vi "Auton Go Backwards.vi"(7 "output range":cluster{"output high":dbl, "output low":dbl}, 9 "Goal":dbl, 10 "PID setpoint":dbl, 11 "Average gains":T1) -> (2 "Done?":bool)   [LabVIEW 2014]
uses:
  DriveGlobal.vi
  Robot Values.vi
  <vilib>/addons/control/pid/pid.llb/PID (DBL).vi
  <vilib>/addons/control/pid/NI_PID_pid.lvlib
panel:
  in  "Diffrence gains":T1={"proportional gain (Kc)"=0.01, "integral time (Ti, min)"=0.0, "derivative time (Td, min)"=0.0} {"derivative time (Td, min)" format="%.3f"; "integral time (Ti, min)" format="%.3f"; "proportional gain (Kc)" format="%.3f"}
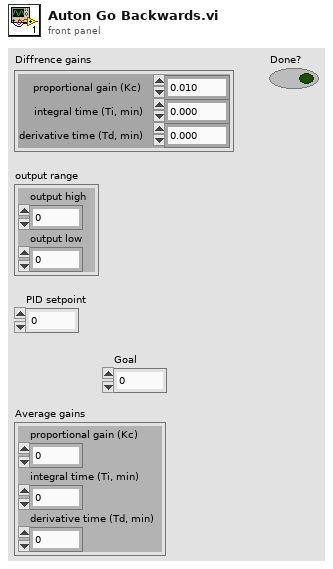
[diagram p1: front panel]
types:
  T1 = cluster{"proportional gain (Kc)":dbl, "integral time (Ti, min)":dbl, "derivative time (Td, min)":dbl}
  T2 = cluster{"Tracking Tote?":bool, "ToteRightSpeed":dbl, "ToteLeftSpeed":dbl, "Drive Encoder reset":bool, "Right Wheel \n(Cm)":dbl, "Left Wheel \n(Cm)":dbl}
  T3 = cluster{"RightMotorSpeed":dbl, "LeftMotorSpeed":dbl}
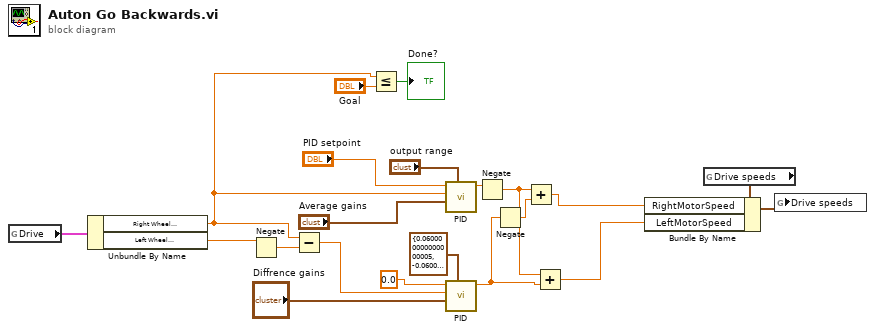
[diagram p0: block diagram]
diagram:
  n1 = global read "Robot Values.vi" "Drive"() -> (w17:T2)
  n2 = Unbundle By Name(w17) -> ("Right Wheel \n(Cm)"=w3:dbl, "Left Wheel \n(Cm)"=w20:dbl)
  n3 = Negate(x=w20) -> (-x=w7:dbl)
  n4 = Subtract(x=w3, y=w7) -> (x-y=w8:dbl)
  n5 = Less Or Equal?(x=w3, y="Goal") -> (x <= y?=→"Done?":bool)
  n6 = call-poly <vilib>:"PID.vi"("output range"="output range", "PID gains"="Average gains", "process variable"=w3, "setpoint"="PID setpoint") -> ("output"=w12:dbl)  [unwired: 6 in, 1 out]
  n7 = call-poly <vilib>:"PID.vi"("output range"=cluster{"output high":dbl, "output low":dbl} {"output high"=0.060000000000000005, "output low"=-0.060000000000000005}, "PID gains"="Diffrence gains", "process variable"=w8, "setpoint"=0.0) -> ("output"=w13:dbl)  [unwired: 6 in, 1 out]
  n8 = Negate(x=w12) -> (-x=w15:dbl)
  n9 = Negate(x=w13) -> (-x=w14:dbl)
  n10 = Add(x=w15, y=w14) -> (x+y=w18:dbl)
  n11 = Add(x=w15, y=w13) -> (x+y=w19:dbl)
  n12 = global read "DriveGlobal.vi" "Drive speeds"() -> (w4:T3)
  n13 = Bundle By Name(cluster=w4, "RightMotorSpeed"=w18, "LeftMotorSpeed"=w19) -> (w5:T3)
  n14 = global write "DriveGlobal.vi" "Drive speeds"(w5) -> ()
